vi "Three Button Dialog.vi"(4 "Allow user to close window? (TRUE)":bool=TRUE, 5 "Justify Message (Left)":enum16{"Left", "Center", "Right"}(ring), 6 "Keyboard Shortcuts (Left is <Enter>)":T2={"Left Button Key Shortcut"={"Control"=FALSE, "Shift"=FALSE, "Key"="<Enter>"}, "Center Button Key Shortcut"={"Control"=FALSE, "Shift"=FALSE, "Key"=""}, "Right Button Key Shortcut"={"Control"=FALSE, "Shift"=FALSE, "Key"=""}}, 7 "Window Title (\"\")":string, 8 "Right Button Text (\"Cancel\")":string="Cancel", 9 "Center Button Text (\"No\")":string="No", 10 "Left Button Text (\"Yes\")":string="Yes", 11 "message":string) -> (3 "Which Button?":T1(ring)=enum."Center Button")   [LabVIEW 2011]
doc: "Displays a dialog box that contains a message and three buttons."
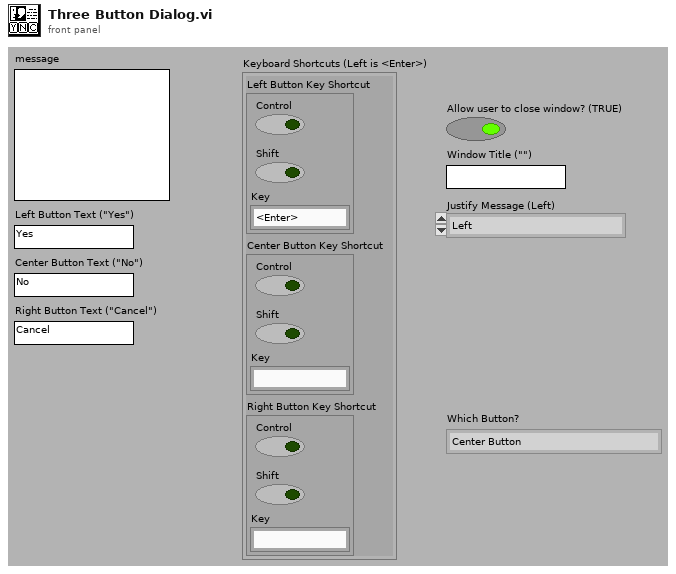
[diagram p1: front panel]
types:
  T1 = enum16{"Left Button", "Center Button", "Right Button", "Window Close"}
  T2 = cluster{"Left Button Key Shortcut":cluster{"Control":bool, "Shift":bool, "Key":string}, "Center Button Key Shortcut":cluster{"Control":bool, "Shift":bool, "Key":string}, "Right Button Key Shortcut":cluster{"Control":bool, "Shift":bool, "Key":string}}
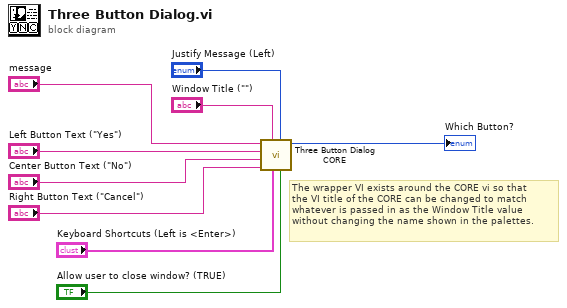
[diagram p0: block diagram]
diagram:
  # "The wrapper VI exists around the CORE vi so that\nthe VI title of the CORE can be changed to match\nwhatever is passed in as the Window Title value\nwithout changing the name shown in the palettes."
  n1 = call "Three Button Dialog CORE.vi"("Allow user to close window? (TRUE)"="Allow user to close window? (TRUE)", "Justify Message (Left)"="Justify Message (Left)", "Keyboard Shortcuts (Left is <Enter>)"="Keyboard Shortcuts (Left is <Enter>)", "Window Title (\"\")"="Window Title (\"\")", "Right Button Text (\"Cancel\")"="Right Button Text (\"Cancel\")", "Center Button Text (\"No\")"="Center Button Text (\"No\")", "Left Button Text (\"Yes\")"="Left Button Text (\"Yes\")", "message"="message") -> ("Which Button?"=→"Which Button?":T1)  [unwired: 3 out]
